vi "Personality Test State.vi"(0 "GEA2 Reference Out in":refnum<k24>, 5 "Queue in":refnum<queue>, 9 "Test Results in":T1, 11 "error in (no error)":errorcluster) -> (4 ".NET Refnum out":refnum<k24>, 10 "Test Results out":T1, 15 "error out":errorcluster)   [LabVIEW 2016]
doc: "This VI performs the personality test state."
uses:
  controls/Test Results.ctl
  C:/Program Files (x86)/National Instruments/LabVIEW 2016/examples/Design Patterns/Queued Message Handler/support/QMH Fundamentals - Message Cluster.ctl
  C:/Automation/DLLs/PC Dot Net/GeaCommunication.dll
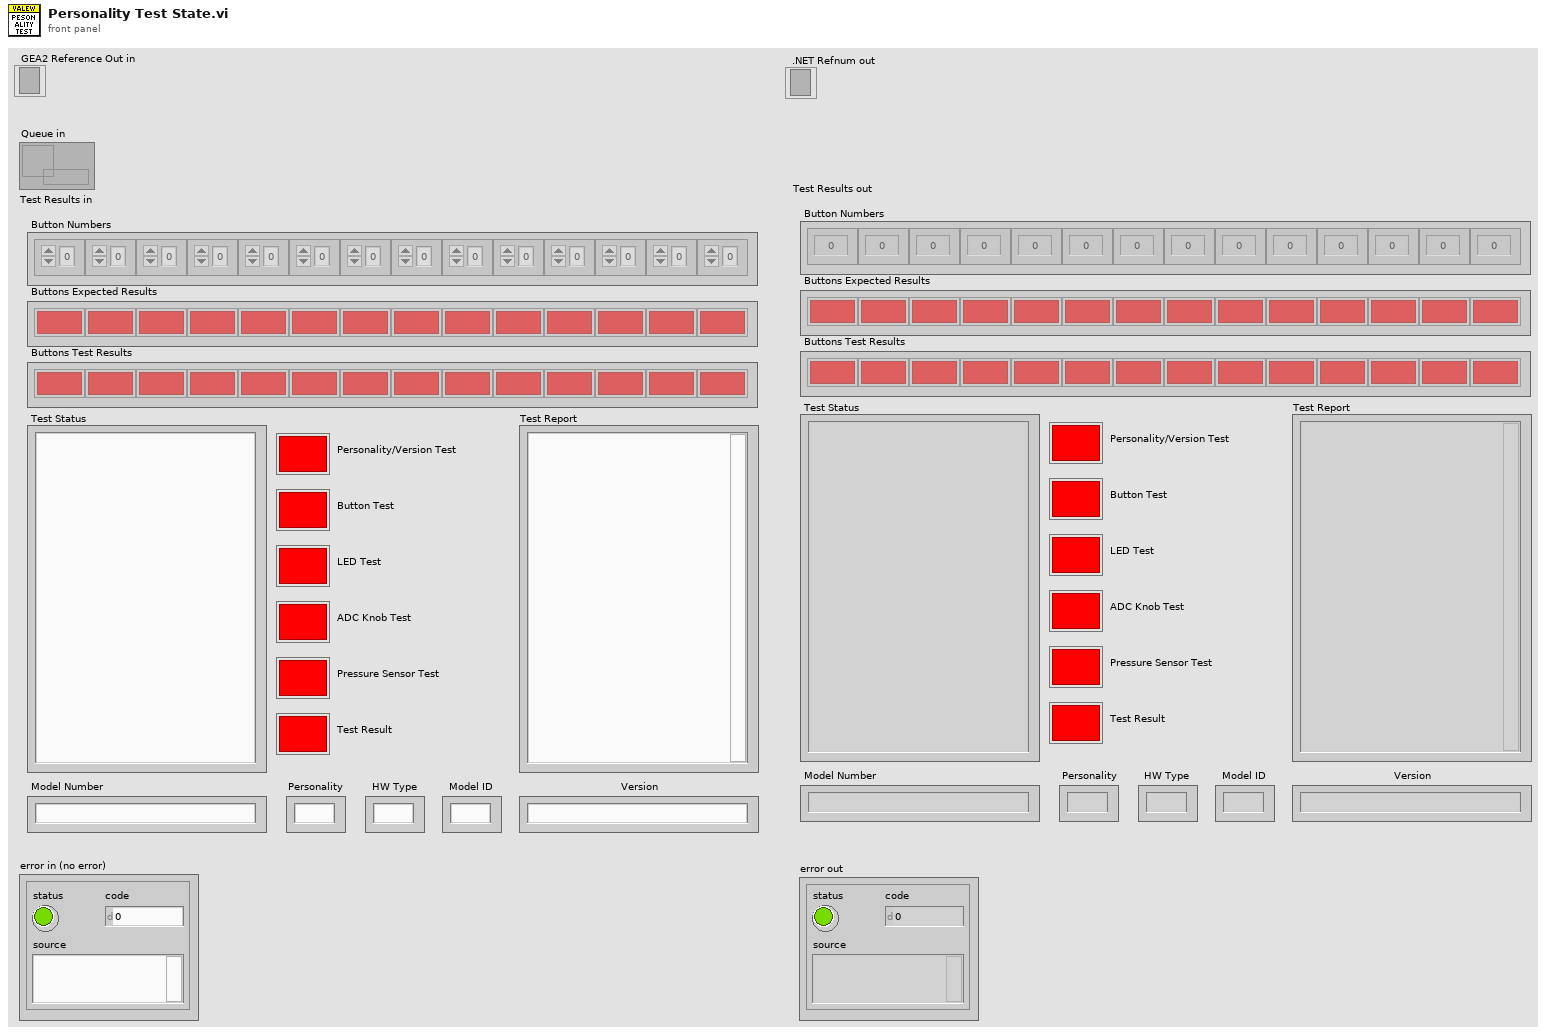
[diagram p1: front panel]
types:
  T1 = typedef "Test Results.ctl" = cluster{"Test Status":string, "Personality/Version Test ":bool, "Test Report":string, "Model Number":string, "Button Numbers":i32[], "Buttons Test Results":bool[], "Buttons Expected Results":bool[], "Model ID":string, "Personality":string, "HW Type":string, "Version":string, "Button Test":bool, "LED Test":bool, "ADC Knob Test":bool, "Pressure Sensor Test":bool, "Test Result":bool}
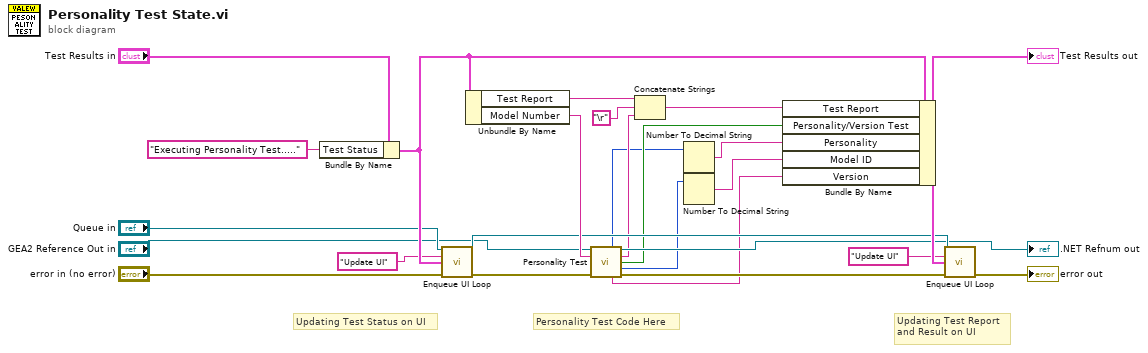
[diagram p0: block diagram]
diagram:
  # "Updating Test Report\nand Result on UI"
  # "Personality Test Code Here"
  # "Updating Test Status on UI"
  n1 = Bundle By Name(cluster="Test Results in", "Test Status"="Executing Personality Test.....") -> (w19:T1)
  n2 = call "Enqueue UI Loop.vi"("UI Que In"="Queue in", "Message"="Update UI", "Test Results"=w19, "error in (no error)"="error in (no error)") -> ("UI Queue Out"=w22:refnum<queue>, "error out"=w16:errorcluster)  [unwired: 10 in]
  n3 = Unbundle By Name(w19) -> ("Test Report"=w9:string, "Model Number"=w25:string)
  n4 = call "Personality Test.vi"("GEA2 Reference In"="GEA2 Reference Out in", "Model"=w25, "error in (no error)"=w16) -> ("Personality"=w5:u8, "GEA2 Reference Out"=→".NET Refnum out":refnum<k24>, "Report Text"=w11:string, "Pass/Fail?"=w7:bool, "Model ID"=w2:u8, "Version"=w1:string, "Error Out"=w20:errorcluster)  [unwired: 6 in]
  n5 = Concatenate Strings(w9, "\r", w11) -> (w10:string)
  n6 = Number To Decimal String(number=w5) -> (decimal integer string=w4:string)  [unwired: 1 in]
  n7 = Number To Decimal String(number=w2) -> (decimal integer string=w3:string)  [unwired: 1 in]
  n8 = Bundle By Name(cluster=w19, "Test Report"=w10, "Personality/Version Test"=w7, "Personality"=w4, "Model ID"=w3, "Version"=w1) -> (w24:T1)
  "Test Results out" <- w24
  n9 = call "Enqueue UI Loop.vi"("UI Que In"=w22, "Message"="Update UI", "Test Results"=w24, "error in (no error)"=w20) -> ("error out"=→"error out":errorcluster)  [unwired: 10 in, 1 out]
